vi "SLSC Create Command Path String.vi"(10 "Physical Channel":string, 11 "name":string) -> (3 "SLSC Path String":string)   [LabVIEW 2015, in "SLSC CD Shared.lvlib"]
uses:
  SLSC CD Shared.lvlib
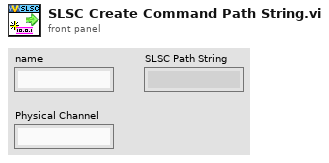
[diagram p1: front panel]
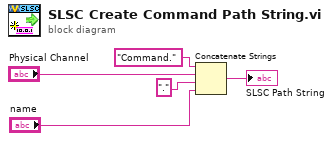
[diagram p0: block diagram]
diagram:
  n1 = Concatenate Strings("Command." ("string"), "Physical Channel", "." ("string"), "name") -> (→"SLSC Path String":string)
